vi "new average.vi"(10 "Numeric 3":dbl, 11 "Numeric in":dbl) -> (3 "Numeric out":dbl)   [LabVIEW 2015]
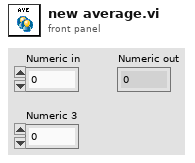
[diagram p1: front panel]
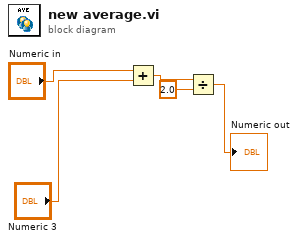
[diagram p0: block diagram]
diagram:
  n1 = Add(x="Numeric in", y="Numeric 3") -> (x+y=w3:dbl)
  n2 = Divide(x=w3, y=2.0) -> (x/y=→"Numeric out":dbl)
